vi "BASIC_test.vi"() -> (2 "Numeric":i32)   [LabVIEW 2015]
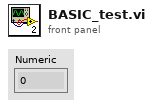
[diagram p1: front panel]
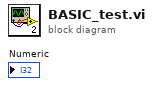
[diagram p0: block diagram]
diagram:
